vi "Disable_Zone_Tuning.vi"   [LabVIEW 2019]
uses:
  Instrument_Setup.vi
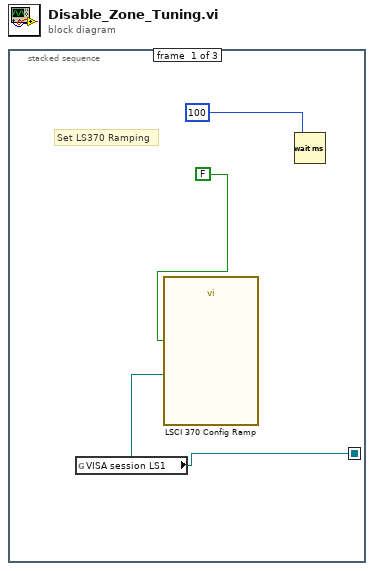
[diagram p0: block diagram]
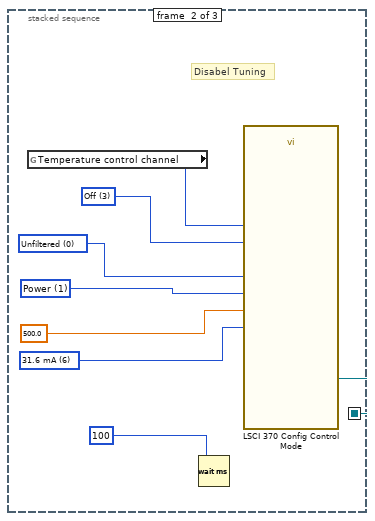
[diagram p2: hidden frame]
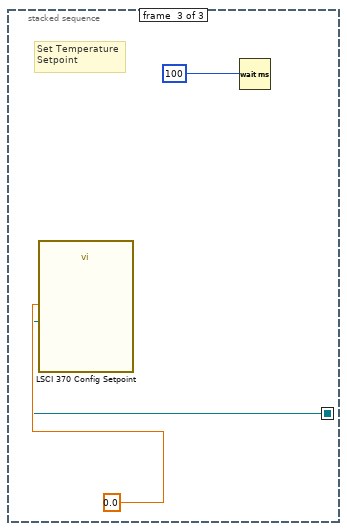
[diagram p3: hidden frame]
diagram:
  n1 = stacked-sequence {
    seq-local: [w1 _ _] -> [_ w5 _]
    seq-local: [_ w5 _] -> [_ _ w12]
    frame #0 {
      # "Set LS370 Ramping"
      n2 = global read "Instrument_Setup.vi" "VISA session LS1"() -> (w1:refnum<visa-resource-name>)
      n3 = call "LSCI 370 Config Ramp.vi"("VISA session"=w1, "Ramping On/Off (F: Ramping Off)"=FALSE) -> ()  [unwired: 12 in, 2 out]
      n4 = Wait (ms)(milliseconds to wait=100) -> ()  [unwired: 1 out]
    }
    frame #1 {
      w11 = u16 6 items=["31.6 uA", "100 uA", "316 uA", "1.00 mA", "3.16 mA", "10.0 mA", "31.6 mA", "100 mA"] ("Maximum Heater Range (0: 31.6 uA)")
      w9 = u16 1 items=["Current", "Power"] ("Heater Output Display (0: Current)")
      w8 = u16 0 items=["Unfiltered", "Filtered"] ("Filtered Readings (0: Unfiltered)")
      w7 = u16 3 items=["Closed Loop PID", "Zone Tuning", "Open Loop", "Off"] ("Control Mode (0: Closed Loop PID)")
      # "Disabel Tuning"
      n5 = global read "Instrument_Setup.vi" "Temperature control channel"() -> (w6:i32)
      n6 = Wait (ms)(milliseconds to wait=100) -> ()  [unwired: 1 out]
      n7 = call "LSCI 370 Config Control Mode.vi"("VISA session"=w5, "Control Mode (0: Closed Loop PID)"=w7, "Channel (1)"=w6, "Filtered Readings (0: Unfiltered)"=w8, "Heater Output Display (0: Current)"=w9, "Heater Resistance (100.00)"=500.0, "Maximum Heater Range (0: 31.6 uA)"=w11) -> ()  [unwired: 7 in, 2 out]
    }
    frame #2 {
      # "Set Temperature\nSetpoint"
      n8 = call "LSCI 370 Config Setpoint.vi"("VISA session"=w12, "Setpoint (0.00000E+0)"=0.0 ("Setpoint")) -> ()  [unwired: 12 in, 2 out]
      n9 = Wait (ms)(milliseconds to wait=100) -> ()  [unwired: 1 out]
    }
  }
